vi "NoServicesRegistered_InvalidRegisterRequests_Error.vi"() -> (6 "Pass":bool, 15 "error out":errorcluster)   [LabVIEW 2020]
uses:
  Discovery Client_lv/Discovery_client/RPC Messages/ni_measurementlink_discovery_v1_RegisterServiceRequest.ctl
  Discovery Client_lv/Discovery_client/RPC Messages/ni_measurementlink_discovery_v1_ServiceDescriptor.ctl
  Discovery Client_lv/Discovery_client/RPC Messages/ni_measurementlink_discovery_v1_ServiceLocation.ctl
  <vilib>/ErrorRing/Error Ring.xnode
  Discovery Client_lv/Discovery_client/Discovery_client.lvlib
panel:
  out "Empty insecure_port fails (as expected)?":bool
  out "Empty display_name fails (as expected)?":bool
  out "Empty location fails (as expected)?":bool
  out "Empty service_class fails (as expected)?":bool
  out "Empty provided_interfaces fails (as expected)?":bool
  # "Test assumes discovery service has already been started."
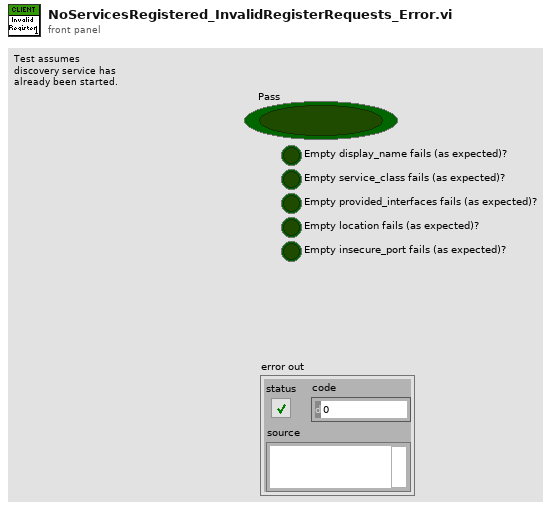
[diagram p1: front panel]
types:
  T1 = typedef "Discovery_client.lvlib/ni_measurementlink_discovery_v1_RegisterServiceRequest.ctl" = cluster{"service_description":T2, "location":T3}
  T2 = typedef "Discovery_client.lvlib/ni_measurementlink_discovery_v1_ServiceDescriptor.ctl" = cluster{"display_name":string, "description_url":string, "provided_interfaces":string[], "service_class":string, "attributes":string[]}
  T3 = typedef "Discovery_client.lvlib/ni_measurementlink_discovery_v1_ServiceLocation.ctl" = cluster{"location":string, "insecure_port":string, "ssl_authenticated_port":string}
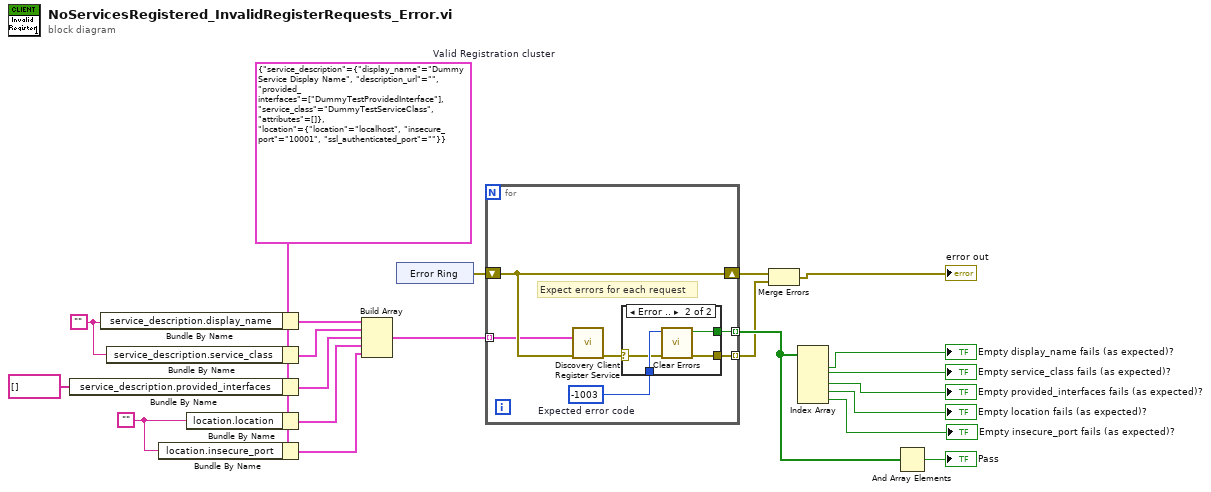
[diagram p0: block diagram]
diagram:
  w6 = ""
  w11 = ""
  w5 = T1 {"service_description"={"display_name"="Dummy Service Display Name", "description_url"="", "provided_interfaces"=["DummyTestProvidedInterface"], "service_class"="DummyTestServiceClass", "attributes"=[]}, "location"={"location"="localhost", "insecure_port"="10001", "ssl_authenticated_port"=""}}  # Valid Registration cluster
  n1 = Bundle By Name(cluster=w5, "service_description.provided_interfaces"=string[] []) -> (w9:T1)
  n2 = Bundle By Name(cluster=w5, "service_description.display_name"=w11) -> (w12:T1)
  n3 = Bundle By Name(cluster=w5, "service_description.service_class"=w11) -> (w10:T1)
  n4 = Bundle By Name(cluster=w5, "location.insecure_port"=w6) -> (w4:T1)
  n5 = Bundle By Name(cluster=w5, "location.location"=w6) -> (w7:T1)
  n6 = Build Array(w12, w10, w9, w7, w4) -> (w13:T1[])
  n7 = xnode "Error Ring"() -> ("error out"=w14:errorcluster)
  n8 = for {
    tunnel: [w25] -> w16 mode=indexing
    tunnel: w13 -> [w26] mode=indexing
    shift-right: [w27] -> w3
    shift-left: w14 -> [w27]
    tunnel: [w24] -> w1 mode=indexing
    w23 = -1003  # Expected error code
    # "Expect errors for each request"
    n9 = call "Discovery Client Register Service.vi"("Request Data"=w26, "error in (no error)"=w27) -> ("error out"=w22:errorcluster)  [unwired: 12 in, 1 out]
    n10 = case shown="Error .." w22 {
      selector: w22 -> [w28 w29]
      tunnel: [_ w32] -> w25
      tunnel: [w28 w31] -> w24
      tunnel: w23 -> [_ w30]
      frame No Error {
      }
      frame Error {
        n11 = call <vilib>:"Clear Errors.vi"("error in (no error)"=w29, "specific error code to clear (0: all)"=w30) -> ("error out"=w31:errorcluster, "specific error cleared?"=w32:bool)  [unwired: 4 in]
      }
    }
  }
  n12 = Merge Errors(w3, w1) -> (→"error out":errorcluster)
  n13 = Index Array(array=w16) -> (element #1=→"Empty display_name fails (as expected)?":bool, element #2=→"Empty service_class fails (as expected)?":bool, element #3=→"Empty provided_interfaces fails (as expected)?":bool, element #4=→"Empty location fails (as expected)?":bool, element #5=→"Empty insecure_port fails (as expected)?":bool)  [unwired: 5 in]
  n14 = And Array Elements(Boolean array=w16) -> (logical AND=→"Pass":bool)
